vi "Perform USB Compliance Autosetup.vi"(8 "error in (no error)":errorcluster, 11 "VISA resource name":refnum<visa-resource-name>) -> (0 "error out":errorcluster, 3 "VISA resource name out":refnum<visa-resource-name>)   [LabVIEW 2015, in "Agilent 2000 3000 X-Series.lvlib"]
doc: "Performs automatic setup of the oscilloscope for the selected\nsignal quality test and USB compliance test packets.\nAutomatically set are:\n- Horizontal scale and delay.\n- Analog input channel(s) scale and vertical offset.\n- Trigger mode and trigger level.\n\nNote:\nThis VI is not supported by EDUX1052A/G, DSOX1202A/G, DSOX1204A/G models."
uses:
  Agilent 2000 3000 X-Series.lvlib
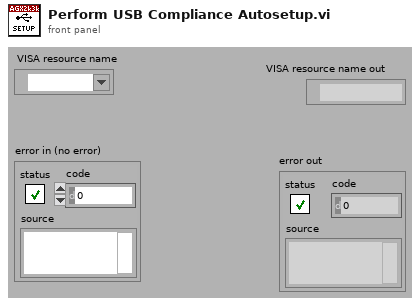
[diagram p1: front panel]
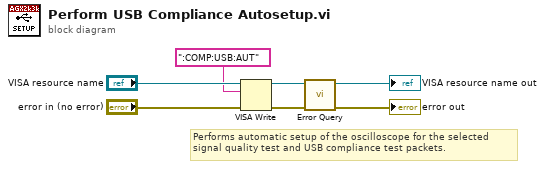
[diagram p0: block diagram]
diagram:
  # "Performs automatic setup of the oscilloscope for the selected\nsignal quality test and USB compliance test packets."
  n1 = VISA Write(VISA resource name="VISA resource name", write buffer=":COMP:USB:AUT", error in (no error)="error in (no error)") -> (VISA resource name out=w3:refnum<visa-resource-name>, error out=w4:errorcluster)  [unwired: 1 out]
  n2 = call "Error Query.vi"("error in (no error)"=w4, "VISA resource name"=w3) -> ("error out"=→"error out":errorcluster, "VISA resource name out"=→"VISA resource name out":refnum<visa-resource-name>)  [unwired: 6 in, 2 out]
